vi "Kill File in RT-Target.vi"(11 "File In":path=path "c:/settings/VOC_DisplayPara.bin") -> ()   [LabVIEW 2024]
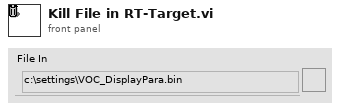
[diagram p1: front panel]
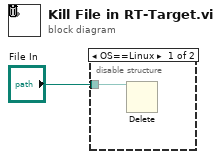
[diagram p0: block diagram]
diagram:
  n1 = disable-structure shown="OS==Linux" {
    disable-tunnel: "File In" -> [w2 _]
    frame condition #0 {
      n2 = Delete(path (use dialog)=w2) -> ()  [unwired: 4 in, 3 out]
    }
    frame condition #1 (active) {
    }
  }
